vi "SVN Checkout Reload.vi"(8 "error in":errorcluster, 9 "ADT version":i32) -> (0 "error out":errorcluster, 1 "SVN Checkout output":string, 2 "commandline":string, 3 "Revision":i32, 4 "Success":bool, 6 "Successful Checkout":bool)   [LabVIEW 2015, in "AguaClara Library.lvlib"]
uses:
  AguaClara Library.lvlib
  mathcad/Simple/MathCAD cmd.ctl
  Word cmd.ctl
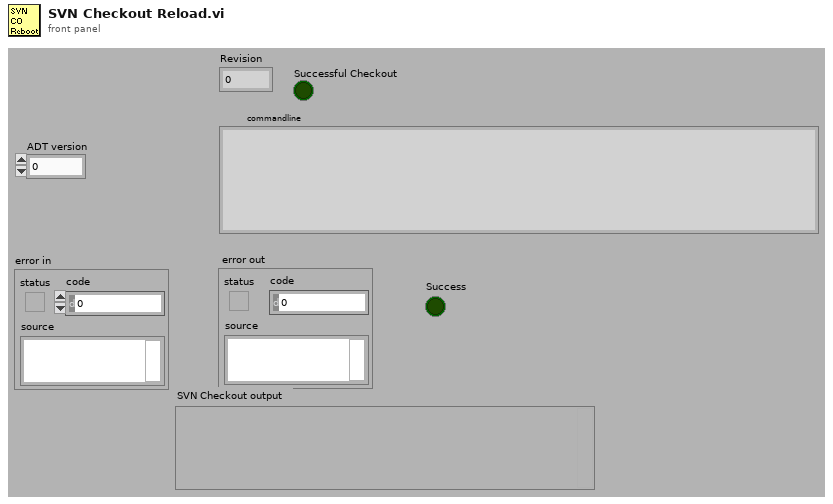
[diagram p1: front panel]
types:
  T1 = typedef "AguaClara Library.lvlib/Word cmd.ctl" = enum16{"Initialize", "Load User Inputs", "Update Fields", "Replace Variables", "Save pdf", "Close Word"}
  T2 = typedef "MathCAD cmd.ctl" = enum16{"Open App", "Open Worksheet", "Close Worksheet", "Load Variable Ref", "Send Number", "Send Cluster", "Send Array", "Send String", "Calculate", "Get MathCAD data", "Close MathCAD"}
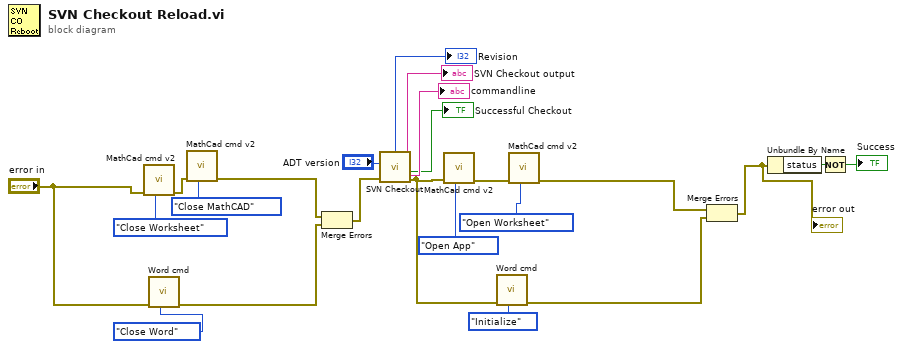
[diagram p0: block diagram]
diagram:
  n1 = call "MathCad cmd v2.vi"("MathCAD cmds"=MathCAD_cmd."Close Worksheet", "error in"="error in") -> ("first error out"=w19:errorcluster)  [unwired: 8 in, 1 out]
  n2 = call "Word cmd.vi"("Word cmd"=Word_cmd."Close Word", "Error In (no error)"="error in") -> ("error out"=w6:errorcluster)  [unwired: 8 in, 1 out]
  n3 = call "MathCad cmd v2.vi"("MathCAD cmds"=MathCAD_cmd."Close MathCAD", "error in"=w19) -> ("first error out"=w5:errorcluster)  [unwired: 8 in, 1 out]
  n4 = Merge Errors(w5, w6) -> (w4:errorcluster)
  n5 = call "SVN Checkout.vi"("error in (no error)"=w4, "ADT version"="ADT version") -> ("error out"=w10:errorcluster, "Successful Checkout"=→"Successful Checkout":bool, "Revision"=→"Revision":i32, "standard output"=→"SVN Checkout output":string, "commandline"=→"commandline":string)  [unwired: 5 in]
  n6 = call "MathCad cmd v2.vi"("MathCAD cmds"=MathCAD_cmd."Open App", "error in"=w10) -> ("first error out"=w21:errorcluster)  [unwired: 8 in, 1 out]
  n7 = call "Word cmd.vi"("Word cmd"=Word_cmd."Initialize", "Error In (no error)"=w10) -> ("error out"=w9:errorcluster)  [unwired: 8 in, 1 out]
  n8 = call "MathCad cmd v2.vi"("MathCAD cmds"=MathCAD_cmd."Open Worksheet", "error in"=w21) -> ("first error out"=w1:errorcluster)  [unwired: 8 in, 1 out]
  n9 = Merge Errors(w1, w9) -> (w8:errorcluster)
  "error out" <- w8
  n10 = Unbundle By Name(w8) -> ("status"=w13:bool)
  n11 = Not(x=w13) -> (.not. x?=→"Success":bool)
